vi "Deom.vi"(2 "error in (no error)":errorcluster) -> (0 "error out":errorcluster, 3 "set IRPower in W":string)   [LabVIEW 2011]
uses:
  <vilib>/DAQmx/read.llb/DAQmx Read (Analog DBL 1Chan 1Samp).vi
  <vilib>/DAQmx/miscellaneous.llb/DAQmx Fill In Error Info.vi
panel:
  out "Waveform Graph":dbl[][](graph)
  out "Waveform Chart":cluster{"mW to serach":dbl, dbl}(graph)
  out "Found Diode":dbl
  out "search PD":dbl
  in  "Set Bias Voltage\nSee FrontPanel: -300V":dbl=-300.0
  out "Found mW":dbl=27.59081560595219
  out "Iteration":i32=3
  out "nm":dbl=751.0
  out "mW to serach":dbl=26.516448089513062
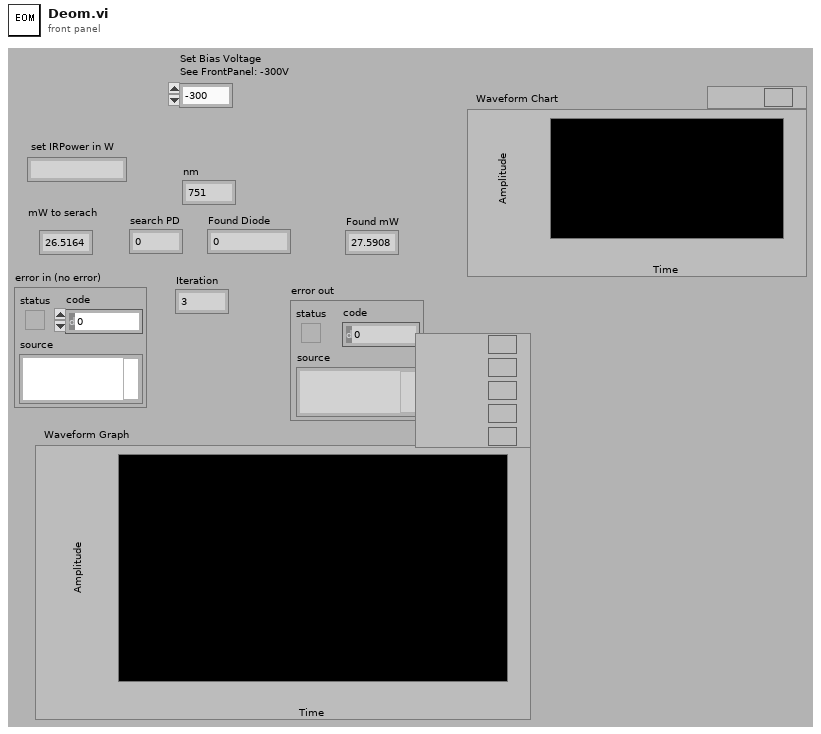
[diagram p1: front panel]
types:
  T1 = enum16{"None/#Datasets", "Clear", "TagValueOf#", "AddValues", "ReadValue", "ChangeValue", "Get all"}
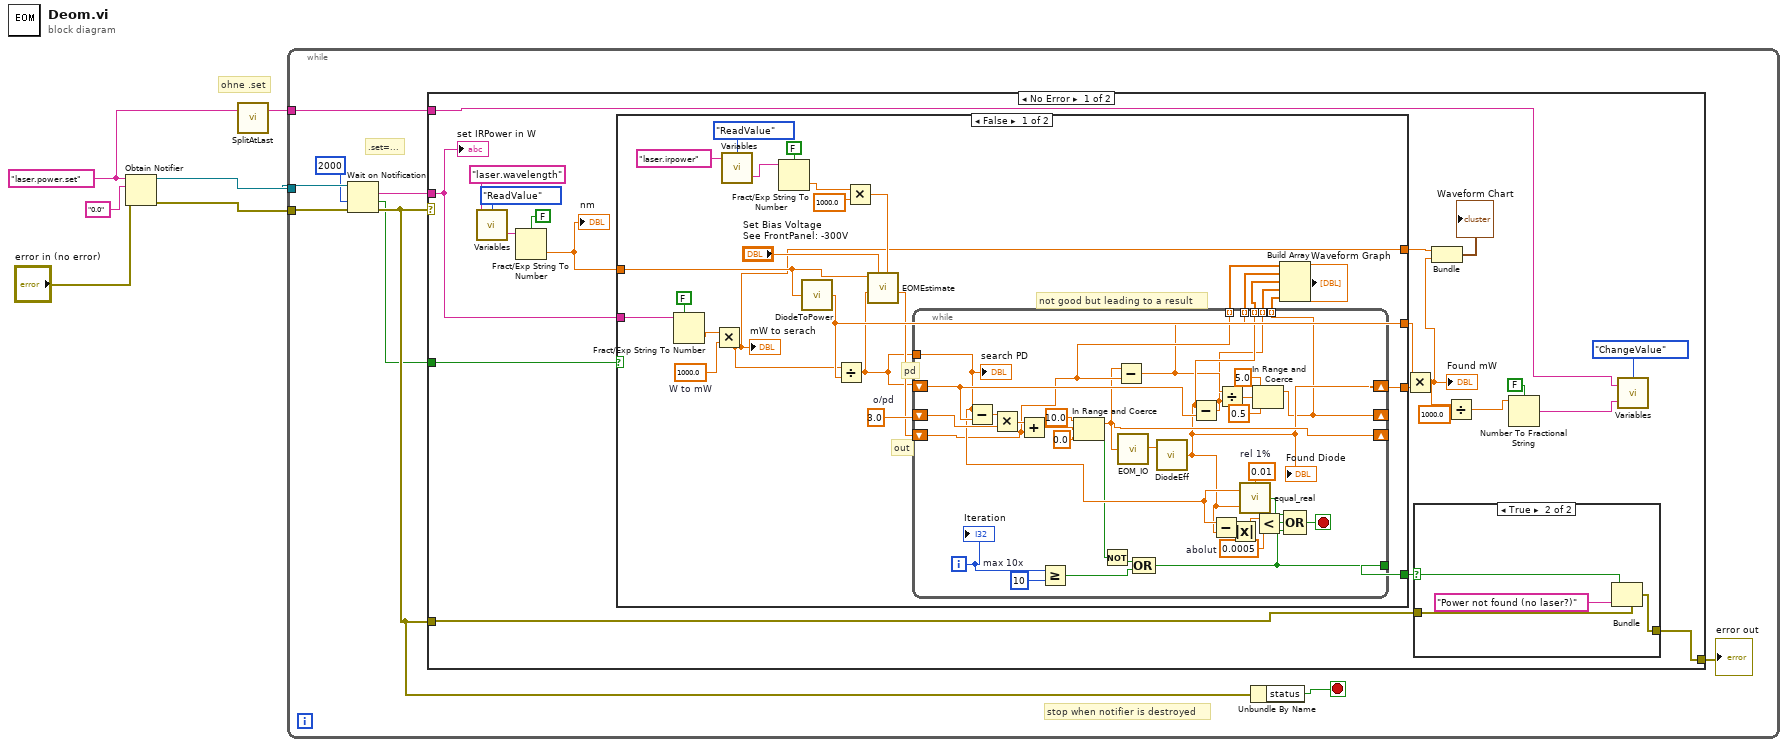
[diagram p0: block diagram]
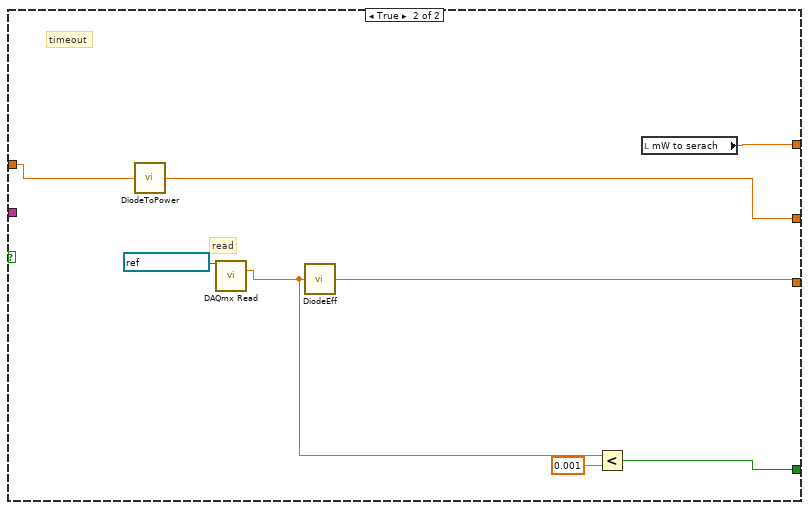
[diagram p2: hidden frame]
diagram:
  w2 = "laser.power.set" ("name (unnamed)")
  # "ohne .set"
  n1 = Obtain Notifier(name (unnamed)=w2, notification data type="0.0", error in (no error)="error in (no error)") -> (notifier out=w5:refnum<notifier>, error out=w3:errorcluster)  [unwired: 1 in, 1 out]
  n2 = call "SplitAtLast.vi"("In-String"=w2) -> ("Front (default)"=w1:string)  [unwired: 1 in, 1 out]
  n3 = while {
    tunnel: w5 -> [w14]
    tunnel: w3 -> [w13]
    tunnel: w1 -> [w7]
    stop <- w10 stop-if-true
    # "stop when notifier is destroyed"
    # ".set=..."
    n4 = Wait on Notification(notifier=w14, timeout in ms (-1)=2000, error in (no error)=w13) -> (notification=w12:string, timed out?=w9:bool, error out=w11:errorcluster)  [unwired: 2 out]
    n5 = case shown="No Error" w11 {
      tunnel: [w29 w107] -> w15
      tunnel: w11 -> [w28 w107]
      tunnel: w12 -> [w21 _]
      tunnel: w9 -> [w22 _]
      tunnel: w7 -> [w20 _]
      frame No Error {
        n6 = call "Variables.vi"("Tag in"="laser.wavelength", "Command"=T1."ReadValue") -> ("value out"=w33:string)  [unwired: 1 in, 2 out]
        n7 = Fract/Exp String To Number(use system decimal point (T)=FALSE, string=w33) -> (number=w32:dbl)  [unwired: 3 out]
        "nm" <- w32
        n8 = case shown="False" w22 {
          tunnel: [w61 w99] -> w36
          tunnel: [w60 w98] -> w19
          tunnel: w32 -> [w56 w101]
          tunnel: [w55 w95] -> w30
          tunnel: w21 -> [w44 _]
          tunnel: [w43 w94] -> w17
          frame False {
            w52 = 1000.0  # W to mW
            w62 = 3.0  # o/pd
            # "not good but leading to a result"
            # "pd"
            # "out"
            n9 = Fract/Exp String To Number(use system decimal point (T)=FALSE, string=w44) -> (number=w53:dbl)  [unwired: 3 out]
            n10 = Multiply(x=w53, y=w52) -> (x*y=w43:dbl)
            "mW to serach" <- w43
            n11 = call "Variables.vi"("Tag in"="laser.irpower", "Command"=T1."ReadValue") -> ("value out"=w48:string)  [unwired: 1 in, 2 out]
            n12 = Fract/Exp String To Number(use system decimal point (T)=FALSE, string=w48) -> (number=w47:dbl)  [unwired: 3 out]
            n13 = call "DiodeToPower.vi"("nm"=w56) -> ("mW/Volt"=w60:dbl)
            n14 = Divide(x=w43, y=w60) -> (x/y=w57:dbl)
            n15 = Multiply(x=w47, y=1000.0) -> (x*y=w45:dbl)
            n16 = call "EOMEstimate.vi"("PD"=w57, "nm"=w56, "Bias Voltage (-200)"="Set Bias Voltage\nSee FrontPanel: -300V", "LaserIR [mW]\n<0: estimate"=w45) -> ("Vestimate"=w58:dbl)  [unwired: 1 in, 6 out]
            n17 = while {
              shift-right: [w67] -> _
              shift-left: w58 -> [w68]
              tunnel: w57 -> [w84]
              shift-right: [w65] -> _
              shift-left: w62 -> [w92]
              shift-right: [w66] -> w61
              shift-left: w57 -> [w90]
              tunnel: [w69] -> w55
              tunnel: [w68] -> w42 mode=indexing
              tunnel: [w64] -> w41 mode=indexing
              tunnel: [w66] -> w40 mode=indexing
              tunnel: [w65] -> w38 mode=indexing
              tunnel: [w63] -> w37 mode=indexing
              i -> [w77]
              stop <- w78 stop-if-true
              w76 = 10  # max 10x
              w81 = 0.0005  # abolut
              w85 = 0.01  # rel 1%
              n18 = Subtract(x=w84, y=w90) -> (x-y=w93:dbl)
              n19 = Multiply(x=w93, y=w92) -> (x*y=w91:dbl)
              n20 = Add(x=w91, y=w68) -> (x+y=w75:dbl)
              n21 = Greater Or Equal?(x=w77, y=w76) -> (x >= y?=w70:bool)
              n22 = In Range and Coerce(upper limit=10.0, x=w75, lower limit=0.0) -> (coerced(x)=w67:dbl, In Range?=w72:bool)
              n23 = Not(x=w72) -> (.not. x?=w71:bool)
              n24 = Subtract(x=w67, y=w68) -> (x-y=w64:dbl)
              n25 = call "EOM_IO.vi"("U_out"=w67) -> ("Diode"=w86:dbl)
              n26 = Compound Arithmetic op=OR(w71, w70) -> (w69:bool)
              n27 = call "DiodeEff.vi"("DiodeU"=w86) -> ("DiodeUeff"=w66:dbl)
              "Found Diode" <- w66
              n28 = Subtract(x=w66, y=w90) -> (x-y=w63:dbl)
              n29 = Subtract(x=w84, y=w66) -> (x-y=w83:dbl)
              n30 = Divide(x=w64, y=w63) -> (x/y=w89:dbl)
              n31 = Absolute Value(x=w83) -> (abs(x)=w82:dbl)
              n32 = call "equal_real.vi"("max rel deviation"=w85, "b"=w66, "a"=w84) -> ("Equal"=w80:bool)
              n33 = In Range and Coerce(upper limit=5.0, x=w89, lower limit=0.5) -> (coerced(x)=w65:dbl)  [unwired: 1 out]
              n34 = Less?(x=w82, y=w81) -> (x < y?=w79:bool)
              n35 = Compound Arithmetic op=OR(w80, w79, w69) -> (w78:bool)
              "Iteration" <- w77
              "search PD" <- w84
            }
            n36 = Build Array(w42, w41, w40, w37, w38) -> (→"Waveform Graph":dbl[][])
          }
          frame True {
            # "timeout"
            # "read"
            n37 = call "DiodeToPower.vi"("nm"=w101) -> ("mW/Volt"=w98:dbl)
            n38 = call-poly <vilib>:"DAQmx Read.vi"("task/channels in"=refnum<k21> "AI0USB_PD") -> ("data"=w97:dbl)  [unwired: 1 in, 13 out]
            n39 = call "DiodeEff.vi"("DiodeU"=w97) -> ("DiodeUeff"=w99:dbl)
            n40 = Less?(x=w97, y=0.001) -> (x < y?=w95:bool)
            n41 = local read "mW to serach"() -> (w94:dbl)
          }
        }
        n42 = Multiply(x=w19, y=w36) -> (x*y=w18:dbl)
        "Found mW" <- w18
        n43 = case shown="True" w30 {
          selector: w30 -> [_ w104]
          tunnel: w28 -> [w102 w106]
          tunnel: [w102 w105] -> w29
          frame False {
          }
          frame True {
            n44 = Bundle(cluster=w106, "status"=w104, "source"="Power not found (no laser?)") -> (w105:errorcluster)  [unwired: 1 out]
          }
        }
        n45 = Bundle("mW to serach"=w17, w18) -> (→"Waveform Chart":cluster{"mW to serach":dbl, dbl})  [unwired: 1 in]
        n46 = Divide(x=w18, y=1000.0) -> (x/y=w24:dbl)
        n47 = Number To Fractional String(use system decimal point (T)=FALSE, number=w24) -> (F-format string=w26:string)  [unwired: 2 out]
        n48 = call "Variables.vi"("value"=w26, "Tag in"=w20, "Command"=T1."ChangeValue") -> ()  [unwired: 3 out]
        "set IRPower in W" <- w21
      }
      frame Error {
      }
    }
    "error out" <- w15
    n49 = Unbundle By Name(w11) -> ("status"=w10:bool)
  }
